vi "Start.vi"(8 "error in (no error)":errorcluster, 10 "Message in":refnum<class "StartMessage.lvclass">, 11 "DAQCascade512II in":refnum<class "DAQCascade512II.lvclass">) -> (0 "error out":errorcluster, 3 "DAQCascade512II out":refnum<class "DAQCascade512II.lvclass">)   [LabVIEW 2012, in "DAQCascade512II.lvclass"]
doc: "This member function is called when the statemachine in the run.vi receives an 'start' command. It relays the message to all observers of the component.\n\nOverride this member function in your derived class if you need additional start functionality (but don't forget to call the parent method)."
uses:
  DAQCascade512II.lvclass
  <vilib>/Distrio/Murmex/StartMessage/StartMessage.lvclass
  <vilib>/Distrio/Murmex/Murmex/Murmex.lvclass
  <vilib>/Distrio/Murmex/StartMessage/run mode enum.ctl
  DAQCascade512II.lvclass/DAQCascade512II.ctl
  <vilib>/Distrio/Murmex/ProceedMessage/ProceedMessage.lvclass
  <vilib>/Distrio/Murmex/StopMessage/StopMessage.lvclass
panel:
  out "Display Title":string
  # "This member function is called when the statemachine in the run.vi receives an 'start' command. It relays the message to all observers of the component.\n\nOverride this member function in your derived class if you need additional start functionality (but don't forget to call the parent method)."
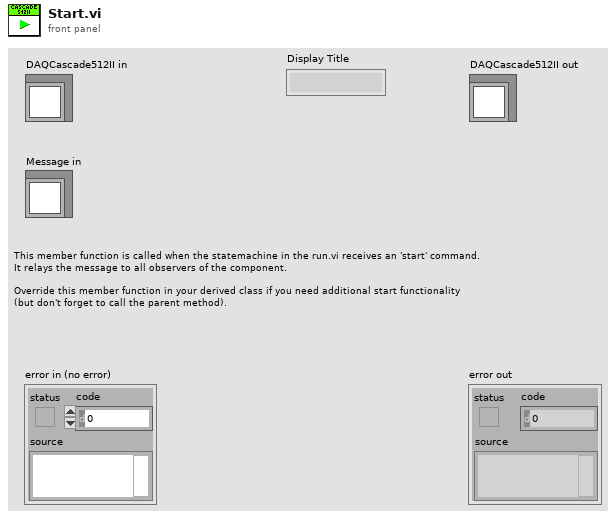
[diagram p1: front panel]
types:
  T1 = typedef "Murmex.lvlib/StartMessage.lvclass/run mode enum.ctl" = enum16{"infinite", "finite"}
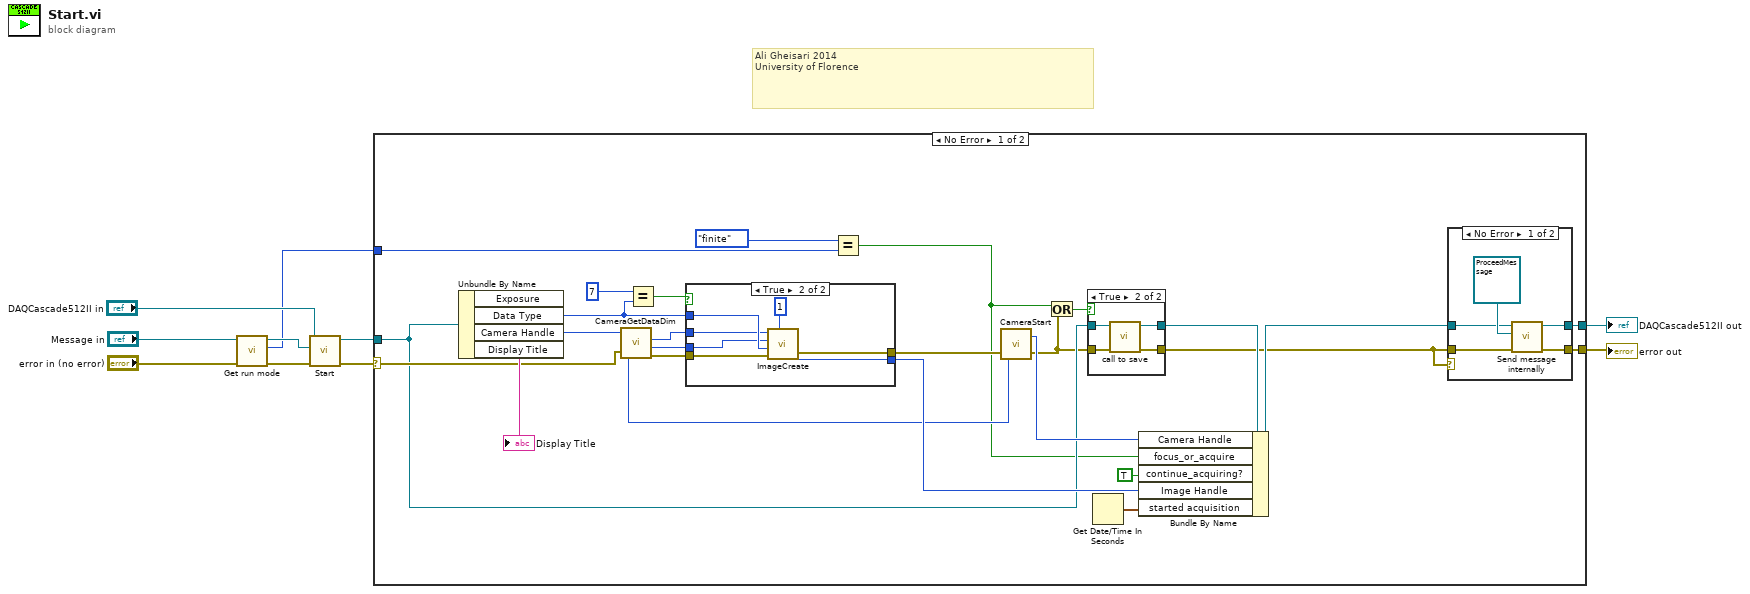
[diagram p0: block diagram]
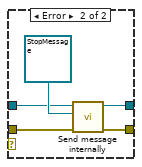
[diagram p3: hidden frame]
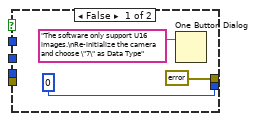
[diagram p4: hidden frame]
diagram:
  # "Ali Gheisari 2014\nUniversity of Florence"
  n1 = call <vilib>:"Get run mode.vi"("error in (no error)"="error in (no error)", "StartMessage in"="Message in") -> ("error out"=w5:errorcluster, "run mode"=w2:T1, "StartMessage out"=w3:refnum<class "StartMessage.lvclass">)  [unwired: 7 in]
  n2 = call-parent "Start.vi"("error in (no error)"=w5, "Message in"=w3, "Murmex in"="DAQCascade512II in") -> ("error out"=w8:errorcluster, "Murmex out"=w7:refnum<class "DAQCascade512II.lvclass">)  [unwired: 7 in]
  n3 = case shown="No Error" w8 {
    selector: w8 -> [w19 w62]
    tunnel: [w35 w63] -> w1
    tunnel: w7 -> [w18 w63]
    tunnel: [w34 w62] -> w6
    tunnel: w2 -> [w31 _]
    frame No Error {
      n4 = Unbundle By Name(w18) -> ("Data Type"=w23:u32, "Camera Handle"=w20:u32, "Display Title"=→"Display Title":string)  [unwired: 1 out]
      n5 = call <userlib>:"CameraGetDataDim.vi"("Camera Handle"=w20, "error in"=w19) -> ("Xdim"=w27:u32, "Ydim"=w28:u32, "error out"=w29:errorcluster)  [unwired: 1 out]
      n6 = Equal?(x=u32 7, y=w23) -> (x = y?=w21:bool)
      n7 = case shown="True" w21 {
        tunnel: w29 -> [_ w61]
        tunnel: w23 -> [_ w60]
        tunnel: w28 -> [_ w59]
        tunnel: w27 -> [_ w58]
        tunnel: [u32 0 ("Image Handle") w57] -> w26
        tunnel: [errorcluster {"status"=TRUE, "code"=1003, "source"="wrong image type"} ("error out") w55] -> w24
        frame False {
          n8 = One Button Dialog(message="The software only support U16 images.\nRe-initialize the camera and choose \"7\" as Data Type") -> ()  [unwired: 1 in, 1 out]
        }
        frame True {
          n9 = call <userlib>:"ImageCreate.vi"("X dimension"=w58, "Y dimension"=w59, "Data Type"=w60, "error in"=w61, "Number Of Frames"=u32 1) -> ("Image Handle"=w57:u32, "error out"=w55:errorcluster)
        }
      }
      n10 = Equal?(x=run_mode_enum."finite" ("run mode"), y=w31) -> (x = y?=w16:bool)
      n11 = call <userlib>:"CameraStart.vi"("error in"=w24, "Camera Handle"=w20) -> ("error out"=w17:errorcluster, "Camera Handle"=w33:u32)
      n12 = Or(x=w16, y=w17) -> (x .or. y?=w15:bool)
      n13 = case shown="True" w15 {
        tunnel: w18 -> [w37 w41]
        tunnel: [w37 w40] -> w13
        tunnel: w17 -> [w36 w39]
        tunnel: [w36 w38] -> w11
        frame False {
        }
        frame True {
          n14 = call-dynamic "call to save.vi"("error in"=w39, "DAQCascade512II"=w41) -> ("error out"=w38:errorcluster, "DAQCascade512II out"=w40:refnum<class "DAQCascade512II.lvclass">)  [unwired: 8 in]
        }
      }
      n15 = Get Date/Time In Seconds() -> (seconds since 1Jan1904=w14:timestamp)
      n16 = Bundle By Name(cluster=w13, "Camera Handle"=w33, "focus_or_acquire"=w16, "continue_acquiring?"=TRUE, "Image Handle"=w26, "started acquisition"=w14) -> (w12:refnum<class "DAQCascade512II.lvclass">)
      n17 = case shown="No Error" w11 {
        tunnel: [w45 w50] -> w35
        tunnel: [w44 w51] -> w34
        tunnel: w12 -> [w43 w48]
        tunnel: w11 -> [w42 w47]
        frame No Error {
          n18 = call <vilib>:"Send message internally.vi"("error in (no error)"=w42, "Message"=refnum<class "ProceedMessage.lvclass"> refnum ("Distrio Murmex 1.5:ProceedMessage"), "Murmex in"=w43) -> ("error out"=w44:errorcluster, "Murmex out"=w45:refnum<class "DAQCascade512II.lvclass">)  [unwired: 7 in]
        }
        frame Error {
          n19 = call <vilib>:"Send message internally.vi"("error in (no error)"=w47, "Message"=refnum<class "StopMessage.lvclass"> refnum ("Distrio Murmex 1.5:StopMessage"), "Murmex in"=w48) -> ("error out"=w51:errorcluster, "Murmex out"=w50:refnum<class "DAQCascade512II.lvclass">)  [unwired: 7 in]
        }
      }
    }
    frame Error {
    }
  }
  "error out" <- w6
  "DAQCascade512II out" <- w1
